vi "Equals Not A Refnum.vi"(11 "Message Dequeuer":refnum<class "Message Dequeuer.lvclass">) -> (2 "Not a refnum?":bool)   [LabVIEW 2020, in "Actor Framework.lvlib" / "Message Dequeuer.lvclass"]
doc: "(<B>Filename</B>: Actor Framework.lvlib:Message Dequeuer.lvclass:Equals Not A Refnum.vi)\n\nChecks whether a message dequeuer reference is equal to Not a Refnum. Unlike the Not a Number/Path/Refnum? function, this function does not check whether a non-zero reference still is valid. Refer to the detailed help for more information."
uses:
  <vilib>/ActorFramework/Message Dequeuer/Message Dequeuer.lvclass
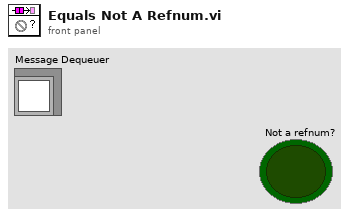
[diagram p1: front panel]
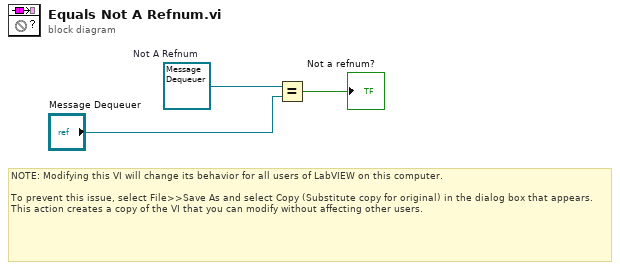
[diagram p0: block diagram]
diagram:
  w3 = refnum<class "Message Dequeuer.lvclass"> refnum  # Not A Refnum
  # "NOTE: Modifying this VI will change its behavior for all users of LabVIEW on this computer.\n\nTo prevent this issue, select File>>Save As and select Copy (Substitute copy for original) in the dialog box that appears. This action creates a copy of the VI that you can modify without affecting other users."
  n1 = Equal?(x=w3, y="Message Dequeuer") -> (x = y?=→"Not a refnum?":bool)
